vi "Connect Core.vi"(4 "queueRef":refnum<queue>, 5 "Commit Only?":bool, 6 "Access (R/W allowed)":T1, 7 "Mode (buffer)":u16(ring)=1 items=["commit", "buffer"], 8 "Error In":errorcluster, 10 "Max Buffer Size":i32, 11 "BNT_SLTagConnection":refnum<class "BNT_SLTagConnection.lvclass">) -> (0 "Error Out":errorcluster, 3 "BNT_SLTagConnection out":refnum<class "BNT_SLTagConnection.lvclass">)   [LabVIEW 2019, in "BNT_SLTagConnection.lvlib" / "BNT_SLTagConnection.lvclass"]
doc: "Open reference to a shared variable if not already connected."
uses:
  BNT_SLTagConnection.lvclass
  C:/Users/Holger/Documents/LVP/CSPP/CSPP-Template/Packages/CSPP_Core/Classes/CSPP_BaseClasses/Base/CSPP_Base.lvclass
  C:/Users/Holger/Documents/LVP/CSPP/CSPP-Template/Packages/CSPP_Core/Classes/CSPP_ProcessVariables/PVConnection/PVConnection.lvclass
  BNT_SLTagConnection.lvclass/BNT_SLTagConnection.ctl
  <vilib>/Skyline/Tag/Wrapper/Wrapper_class/NI Skyline Tag.lvclass/NI Skyline Tag.ctl
  CSPP_Core/Classes/CSPP_BaseClasses/Base/CSPP_Base.lvclass/CSPP_Base.ctl
  CSPP_Core/Classes/CSPP_ProcessVariables/PVConnection/PVConnection.lvclass/PVConnection.ctl
  CSPP_Core/Classes/CSPP_ProcessVariables/ProcessVariable/PV.lvclass/PV.ctl
  CSPP_Core/Libraries/Base/Severity.ctl
  <vilib>/Skyline/Tag/Wrapper/Wrapper_class/Read Tag Path.vi
  CSPP_Core/Classes/CSPP_ProcessVariables/ProcessVariable/PV.lvclass
  <vilib>/Skyline/Tag/Wrapper/Wrapper AMQP_class/Open Tag AMQP.vi
  CSPP_Core/Classes/CSPP_ProcessVariables/PVConnection/PVConnection.lvclass
  CSPP_Core/Libraries/Utilities/CSPP_Utilities.lvlib
  CSPP_Core/Classes/CSPP_BaseClasses/Base/CSPP_Base.lvclass
  CSPP_Core/Libraries/Base/CSPP_Base.lvlib
  <vilib>/Skyline/Tag/Wrapper/Wrapper_class/NI Skyline Tag.lvclass
  BNT_SLTools.lvlib
  <vilib>/Skyline/Tag/Shared/typedefs/DataType.ctl
  <vilib>/Skyline/Tag/Shared/NI Skyline Tag.lvlib
  <vilib>/Skyline/Tag/Wrapper/Wrapper AMQP_class/NI Skyline Tag AMQP.lvclass
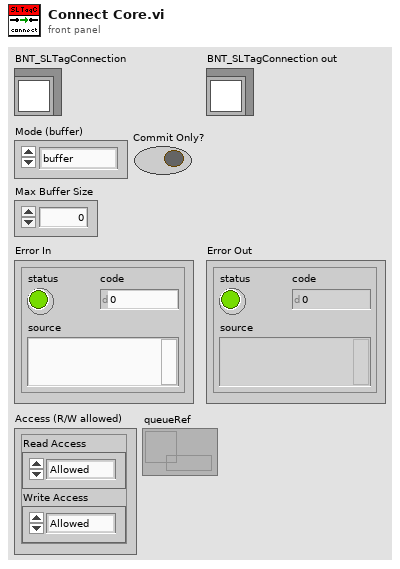
[diagram p1: front panel]
types:
  T1 = cluster{"Read Access":enum8{"Allowed", "Required", "None"}, "Write Access":enum8{"Allowed", "Required", "None"}}
  T2 = typedef "NI Skyline Tag.lvlib/DataType.ctl" = enum32{"Double", "I32", "String", "Boolean", "U64", "Timestamp"}
  T3 = typedef "CSPP_Base.lvlib/Severity.ctl" = enum16{"emergency", "alert", "critical", "error", "warning", "notice", "info", "debug"}
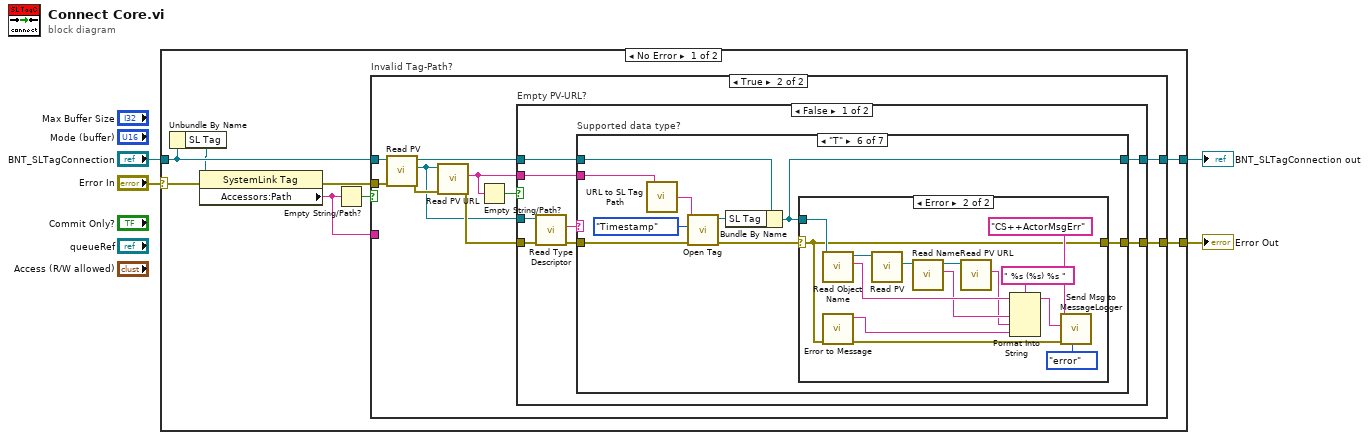
[diagram p0: block diagram]
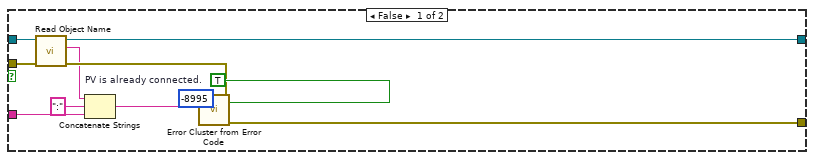
[diagram p2: hidden frame]
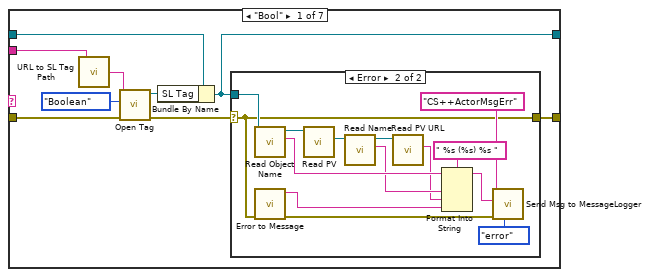
[diagram p3: hidden frame]
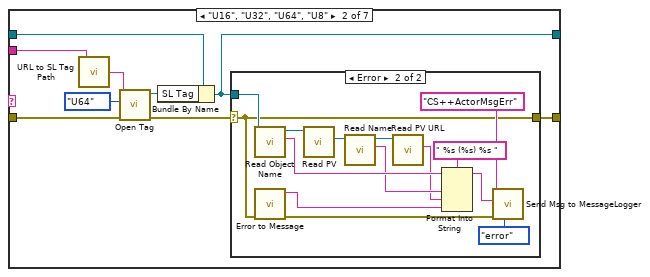
[diagram p5: hidden frame]
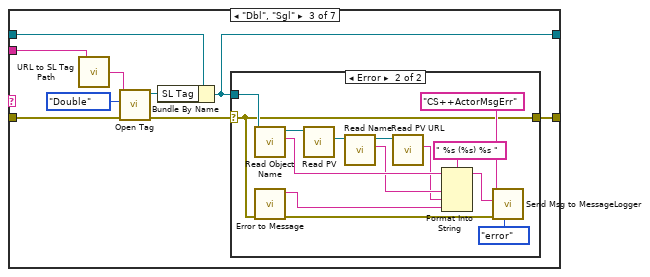
[diagram p7: hidden frame]
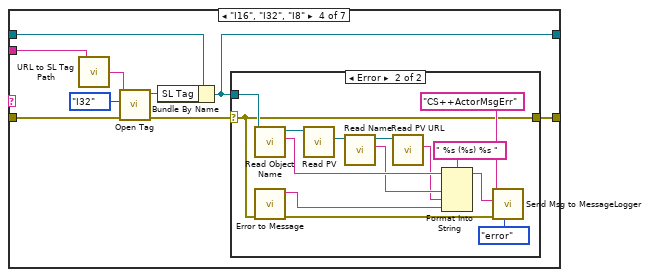
[diagram p9: hidden frame]
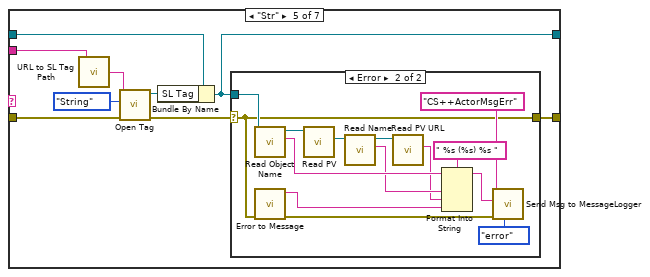
[diagram p11: hidden frame]
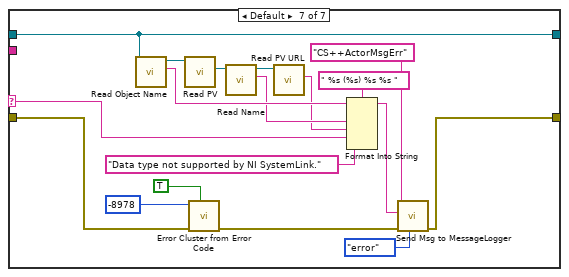
[diagram p14: hidden frame]
diagram:
  n1 = case shown="No Error" "Error In" {
    selector: "Error In" -> [w7 w207]
    tunnel: [w12 w207] -> w3
    tunnel: [w11 w206] -> w1
    tunnel: "BNT_SLTagConnection" -> [w9 w206]
    frame No Error {
      n2 = Unbundle By Name(w9) -> ("SL Tag"=w8:refnum<class "NI Skyline Tag.lvclass">)
      n3 = property class="SystemLink Tag"(reference=w8, error in=w7) -> (error out=w6:errorcluster, "Accessors:Path"=w5:string)  [unwired: 1 out]
      n4 = Empty String/Path?(string/path=w5) -> (empty?=w10:bool)
      n5 = case "Invalid Tag-Path?" shown="True" w10 {
        tunnel: w6 -> [w18 w28]
        tunnel: [w23 w33] -> w12
        tunnel: [w19 w32] -> w11
        tunnel: w9 -> [w20 w31]
        tunnel: w5 -> [w14 _]
        frame False {
          w21 = -8995  # PV is already connected.
          n6 = call "Read Object Name.vi"("error in (no error)"=w18, "Base in"=w20) -> ("error out"=w17:errorcluster, "Object Name"=w16:string, "Base out"=w19:refnum<class "BNT_SLTagConnection.lvclass">)  [unwired: 7 in]
          n7 = Concatenate Strings(w16, ":" ("string"), w14) -> (w13:string)
          n8 = call "Error Cluster from Error Code.vi"("is warning? (False)"=TRUE ("show call chain? (False)"), "Error In"=w17, "Error Message (\"\")"=w13, "Error Code (0)"=w21) -> ("Error Out"=w23:errorcluster)  [unwired: 7 in]
        }
        frame True {
          n9 = call "Read PV.vi"("error in (no error)"=w28, "PVConnection in"=w31) -> ("error out"=w30:errorcluster, "PV"=w24:refnum<class "PV.lvclass">, "PVConnection out"=w25:refnum<class "BNT_SLTagConnection.lvclass">)  [unwired: 7 in]
          n10 = call "Read PV URL.vi"("error in (no error)"=w30, "PV in"=w24) -> ("error out"=w29:errorcluster, "PV URL"=w27:string)  [unwired: 7 in, 1 out]
          n11 = Empty String/Path?(string/path=w27) -> (empty?=w26:bool)
          n12 = case "Empty PV-URL?" shown="False" w26 {
            tunnel: [w40 w205] -> w33
            tunnel: [w41 w204] -> w32
            tunnel: w27 -> [w39 _]
            tunnel: w29 -> [w35 w205]
            tunnel: w25 -> [w38 w204]
            tunnel: w24 -> [w37 _]
            frame False {
              n13 = call "Read Type Descriptor.vi"("error in (no error)"=w35, "PV in"=w37) -> ("error out"=w36:errorcluster, "Type Descriptor"=w34:string)  [unwired: 7 in, 1 out]
              n14 = case "Supported data type?" shown="\"T\"" w34 {
                selector: w34 -> [_ _ _ _ _ _ w186]
                tunnel: [w50 w74 w98 w122 w146 w170 w203] -> w41
                tunnel: [w48 w72 w96 w120 w144 w168 w191] -> w40
                tunnel: w39 -> [w43 w67 w91 w115 w139 w163 _]
                tunnel: w38 -> [w46 w70 w94 w118 w142 w166 w203]
                tunnel: w36 -> [w45 w69 w93 w117 w141 w165 w187]
                frame "Bool" {
                  n15 = call "URL to SL Tag Path.vi"("URL"=w43) -> ("SL Tag Path"=w44:string)
                  n16 = call-poly <vilib>:"Open Tag.vi"("error in (no error)"=w45, "data type"=DataType."Boolean", "path"=w44) -> ("error out"=w49:errorcluster, "tag"=w47:refnum<class "NI Skyline Tag.lvclass">)  [unwired: 7 in]
                  n17 = Bundle By Name(cluster=w46, "SL Tag"=w47) -> (w50:refnum<class "BNT_SLTagConnection.lvclass">)
                  n18 = case shown="Error" w49 {
                    selector: w49 -> [w51 w58]
                    tunnel: w50 -> [_ w60]
                    tunnel: [w51 w58] -> w48
                    frame No Error {
                    }
                    frame Error {
                      n19 = call "Read Object Name.vi"("Base in"=w60) -> ("Object Name"=w59:string, "Base out"=w57:refnum<class "BNT_SLTagConnection.lvclass">)  [unwired: 8 in, 1 out]
                      n20 = call "Error to Message.vi"("Error In"=w58) -> ("Error Out"=w62:errorcluster, "Error Message"=w63:string)  [unwired: 9 in]
                      n21 = call "Read PV.vi"("PVConnection in"=w57) -> ("PV"=w56:refnum<class "PV.lvclass">)  [unwired: 8 in, 2 out]
                      n22 = call "Read Name.vi"("PV in"=w56) -> ("Name"=w54:string, "PV out"=w55:refnum<class "PV.lvclass">)  [unwired: 8 in, 1 out]
                      n23 = call "Read PV URL.vi"("PV in"=w55) -> ("PV URL"=w53:string)  [unwired: 8 in, 2 out]
                      n24 = Format Into String(format string=" %s (%s) %s ", initial string=w59, w54, w53, w63) -> (resulting string=w65:string)  [unwired: 1 in, 1 out]
                      n25 = call "Send Msg to MessageLogger.vi"("Severity Code (info)"=Severity."error", "Error In"=w62, "Message Content"=w65, "Message Tag"="CS++ActorMsgErr") -> ()  [unwired: 7 in, 1 out]
                    }
                  }
                }
                frame "U16", "U32", "U64", "U8" {
                  n26 = call "URL to SL Tag Path.vi"("URL"=w67) -> ("SL Tag Path"=w68:string)
                  n27 = call-poly <vilib>:"Open Tag.vi"("error in (no error)"=w69, "data type"=DataType."U64", "path"=w68) -> ("error out"=w73:errorcluster, "tag"=w71:refnum<class "NI Skyline Tag.lvclass">)  [unwired: 7 in]
                  n28 = Bundle By Name(cluster=w70, "SL Tag"=w71) -> (w74:refnum<class "BNT_SLTagConnection.lvclass">)
                  n29 = case shown="Error" w73 {
                    selector: w73 -> [w75 w82]
                    tunnel: w74 -> [_ w84]
                    tunnel: [w75 w82] -> w72
                    frame No Error {
                    }
                    frame Error {
                      n30 = call "Read Object Name.vi"("Base in"=w84) -> ("Object Name"=w83:string, "Base out"=w81:refnum<class "BNT_SLTagConnection.lvclass">)  [unwired: 8 in, 1 out]
                      n31 = call "Error to Message.vi"("Error In"=w82) -> ("Error Out"=w86:errorcluster, "Error Message"=w87:string)  [unwired: 9 in]
                      n32 = call "Read PV.vi"("PVConnection in"=w81) -> ("PV"=w80:refnum<class "PV.lvclass">)  [unwired: 8 in, 2 out]
                      n33 = call "Read Name.vi"("PV in"=w80) -> ("Name"=w78:string, "PV out"=w79:refnum<class "PV.lvclass">)  [unwired: 8 in, 1 out]
                      n34 = call "Read PV URL.vi"("PV in"=w79) -> ("PV URL"=w77:string)  [unwired: 8 in, 2 out]
                      n35 = Format Into String(format string=" %s (%s) %s ", initial string=w83, w78, w77, w87) -> (resulting string=w89:string)  [unwired: 1 in, 1 out]
                      n36 = call "Send Msg to MessageLogger.vi"("Severity Code (info)"=Severity."error", "Error In"=w86, "Message Content"=w89, "Message Tag"="CS++ActorMsgErr") -> ()  [unwired: 7 in, 1 out]
                    }
                  }
                }
                frame "Dbl", "Sgl" {
                  n37 = call "URL to SL Tag Path.vi"("URL"=w91) -> ("SL Tag Path"=w92:string)
                  n38 = call-poly <vilib>:"Open Tag.vi"("error in (no error)"=w93, "data type"=DataType."Double", "path"=w92) -> ("error out"=w97:errorcluster, "tag"=w95:refnum<class "NI Skyline Tag.lvclass">)  [unwired: 7 in]
                  n39 = Bundle By Name(cluster=w94, "SL Tag"=w95) -> (w98:refnum<class "BNT_SLTagConnection.lvclass">)
                  n40 = case shown="Error" w97 {
                    selector: w97 -> [w99 w106]
                    tunnel: w98 -> [_ w108]
                    tunnel: [w99 w106] -> w96
                    frame No Error {
                    }
                    frame Error {
                      n41 = call "Read Object Name.vi"("Base in"=w108) -> ("Object Name"=w107:string, "Base out"=w105:refnum<class "BNT_SLTagConnection.lvclass">)  [unwired: 8 in, 1 out]
                      n42 = call "Error to Message.vi"("Error In"=w106) -> ("Error Out"=w110:errorcluster, "Error Message"=w111:string)  [unwired: 9 in]
                      n43 = call "Read PV.vi"("PVConnection in"=w105) -> ("PV"=w104:refnum<class "PV.lvclass">)  [unwired: 8 in, 2 out]
                      n44 = call "Read Name.vi"("PV in"=w104) -> ("Name"=w102:string, "PV out"=w103:refnum<class "PV.lvclass">)  [unwired: 8 in, 1 out]
                      n45 = call "Read PV URL.vi"("PV in"=w103) -> ("PV URL"=w101:string)  [unwired: 8 in, 2 out]
                      n46 = Format Into String(format string=" %s (%s) %s ", initial string=w107, w102, w101, w111) -> (resulting string=w113:string)  [unwired: 1 in, 1 out]
                      n47 = call "Send Msg to MessageLogger.vi"("Severity Code (info)"=Severity."error", "Error In"=w110, "Message Content"=w113, "Message Tag"="CS++ActorMsgErr") -> ()  [unwired: 7 in, 1 out]
                    }
                  }
                }
                frame "I16", "I32", "I8" {
                  n48 = call "URL to SL Tag Path.vi"("URL"=w115) -> ("SL Tag Path"=w116:string)
                  n49 = call-poly <vilib>:"Open Tag.vi"("error in (no error)"=w117, "data type"=DataType."I32", "path"=w116) -> ("error out"=w121:errorcluster, "tag"=w119:refnum<class "NI Skyline Tag.lvclass">)  [unwired: 7 in]
                  n50 = Bundle By Name(cluster=w118, "SL Tag"=w119) -> (w122:refnum<class "BNT_SLTagConnection.lvclass">)
                  n51 = case shown="Error" w121 {
                    selector: w121 -> [w123 w130]
                    tunnel: w122 -> [_ w132]
                    tunnel: [w123 w130] -> w120
                    frame No Error {
                    }
                    frame Error {
                      n52 = call "Read Object Name.vi"("Base in"=w132) -> ("Object Name"=w131:string, "Base out"=w129:refnum<class "BNT_SLTagConnection.lvclass">)  [unwired: 8 in, 1 out]
                      n53 = call "Error to Message.vi"("Error In"=w130) -> ("Error Out"=w134:errorcluster, "Error Message"=w135:string)  [unwired: 9 in]
                      n54 = call "Read PV.vi"("PVConnection in"=w129) -> ("PV"=w128:refnum<class "PV.lvclass">)  [unwired: 8 in, 2 out]
                      n55 = call "Read Name.vi"("PV in"=w128) -> ("Name"=w126:string, "PV out"=w127:refnum<class "PV.lvclass">)  [unwired: 8 in, 1 out]
                      n56 = call "Read PV URL.vi"("PV in"=w127) -> ("PV URL"=w125:string)  [unwired: 8 in, 2 out]
                      n57 = Format Into String(format string=" %s (%s) %s ", initial string=w131, w126, w125, w135) -> (resulting string=w137:string)  [unwired: 1 in, 1 out]
                      n58 = call "Send Msg to MessageLogger.vi"("Severity Code (info)"=Severity."error", "Error In"=w134, "Message Content"=w137, "Message Tag"="CS++ActorMsgErr") -> ()  [unwired: 7 in, 1 out]
                    }
                  }
                }
                frame "Str" {
                  n59 = call "URL to SL Tag Path.vi"("URL"=w139) -> ("SL Tag Path"=w140:string)
                  n60 = call-poly <vilib>:"Open Tag.vi"("error in (no error)"=w141, "data type"=DataType."String", "path"=w140) -> ("error out"=w145:errorcluster, "tag"=w143:refnum<class "NI Skyline Tag.lvclass">)  [unwired: 7 in]
                  n61 = Bundle By Name(cluster=w142, "SL Tag"=w143) -> (w146:refnum<class "BNT_SLTagConnection.lvclass">)
                  n62 = case shown="Error" w145 {
                    selector: w145 -> [w147 w154]
                    tunnel: w146 -> [_ w156]
                    tunnel: [w147 w154] -> w144
                    frame No Error {
                    }
                    frame Error {
                      n63 = call "Read Object Name.vi"("Base in"=w156) -> ("Object Name"=w155:string, "Base out"=w153:refnum<class "BNT_SLTagConnection.lvclass">)  [unwired: 8 in, 1 out]
                      n64 = call "Error to Message.vi"("Error In"=w154) -> ("Error Out"=w158:errorcluster, "Error Message"=w159:string)  [unwired: 9 in]
                      n65 = call "Read PV.vi"("PVConnection in"=w153) -> ("PV"=w152:refnum<class "PV.lvclass">)  [unwired: 8 in, 2 out]
                      n66 = call "Read Name.vi"("PV in"=w152) -> ("Name"=w150:string, "PV out"=w151:refnum<class "PV.lvclass">)  [unwired: 8 in, 1 out]
                      n67 = call "Read PV URL.vi"("PV in"=w151) -> ("PV URL"=w149:string)  [unwired: 8 in, 2 out]
                      n68 = Format Into String(format string=" %s (%s) %s ", initial string=w155, w150, w149, w159) -> (resulting string=w161:string)  [unwired: 1 in, 1 out]
                      n69 = call "Send Msg to MessageLogger.vi"("Severity Code (info)"=Severity."error", "Error In"=w158, "Message Content"=w161, "Message Tag"="CS++ActorMsgErr") -> ()  [unwired: 7 in, 1 out]
                    }
                  }
                }
                frame "T" {
                  n70 = call "URL to SL Tag Path.vi"("URL"=w163) -> ("SL Tag Path"=w164:string)
                  n71 = call-poly <vilib>:"Open Tag.vi"("error in (no error)"=w165, "data type"=DataType."Timestamp", "path"=w164) -> ("error out"=w169:errorcluster, "tag"=w167:refnum<class "NI Skyline Tag.lvclass">)  [unwired: 7 in]
                  n72 = Bundle By Name(cluster=w166, "SL Tag"=w167) -> (w170:refnum<class "BNT_SLTagConnection.lvclass">)
                  n73 = case shown="Error" w169 {
                    selector: w169 -> [w171 w178]
                    tunnel: w170 -> [_ w180]
                    tunnel: [w171 w178] -> w168
                    frame No Error {
                    }
                    frame Error {
                      n74 = call "Read Object Name.vi"("Base in"=w180) -> ("Object Name"=w179:string, "Base out"=w177:refnum<class "BNT_SLTagConnection.lvclass">)  [unwired: 8 in, 1 out]
                      n75 = call "Error to Message.vi"("Error In"=w178) -> ("Error Out"=w182:errorcluster, "Error Message"=w183:string)  [unwired: 9 in]
                      n76 = call "Read PV.vi"("PVConnection in"=w177) -> ("PV"=w176:refnum<class "PV.lvclass">)  [unwired: 8 in, 2 out]
                      n77 = call "Read Name.vi"("PV in"=w176) -> ("Name"=w174:string, "PV out"=w175:refnum<class "PV.lvclass">)  [unwired: 8 in, 1 out]
                      n78 = call "Read PV URL.vi"("PV in"=w175) -> ("PV URL"=w173:string)  [unwired: 8 in, 2 out]
                      n79 = Format Into String(format string=" %s (%s) %s ", initial string=w179, w174, w173, w183) -> (resulting string=w185:string)  [unwired: 1 in, 1 out]
                      n80 = call "Send Msg to MessageLogger.vi"("Severity Code (info)"=Severity."error", "Error In"=w182, "Message Content"=w185, "Message Tag"="CS++ActorMsgErr") -> ()  [unwired: 7 in, 1 out]
                    }
                  }
                }
                frame Default {
                  n81 = call "Read Object Name.vi"("Base in"=w203) -> ("Object Name"=w199:string, "Base out"=w198:refnum<class "BNT_SLTagConnection.lvclass">)  [unwired: 8 in, 1 out]
                  n82 = call "Read PV.vi"("PVConnection in"=w198) -> ("PV"=w197:refnum<class "PV.lvclass">)  [unwired: 8 in, 2 out]
                  n83 = call "Error Cluster from Error Code.vi"("show call chain? (False)"=TRUE, "Error In"=w187, "Error Code (0)"=-8978 ("error code (0)")) -> ("Error Out"=w188:errorcluster)  [unwired: 8 in]
                  n84 = call "Read Name.vi"("PV in"=w197) -> ("Name"=w195:string, "PV out"=w196:refnum<class "PV.lvclass">)  [unwired: 8 in, 1 out]
                  n85 = call "Read PV URL.vi"("PV in"=w196) -> ("PV URL"=w194:string)  [unwired: 8 in, 2 out]
                  n86 = Format Into String(format string=" %s (%s) %s %s ", initial string=w199, w195, w194, w186, "Data type not supported by NI SystemLink." ("input 3")) -> (resulting string=w202:string)  [unwired: 1 in, 1 out]
                  n87 = call "Send Msg to MessageLogger.vi"("Severity Code (info)"=Severity."error", "Error In"=w188, "Message Content"=w202, "Message Tag"="CS++ActorMsgErr") -> ("Error Out"=w191:errorcluster)  [unwired: 7 in]
                }
              }
            }
            frame True {
            }
          }
        }
      }
    }
    frame Error {
    }
  }
  "Error Out" <- w3
  "BNT_SLTagConnection out" <- w1
